vi "Target_9.vi"   [LabVIEW 2020]
uses:
  <vilib>/Platform/TimedLoop/XDataNode/timing_clust.ctl
  <vilib>/Platform/TimedLoop/XDataNode/nitl_modes.ctl
  <vilib>/Platform/TimedLoop/XDataNode/wakeup.ctl
  <vilib>/Platform/TimedLoop/XDataNode/XDataNode.xnode
  <vilib>/Platform/TimedLoop/XDataNode/XDNodeRunTimeDep.lvlib
  <vilib>/measure/NI_MABase.lvlib
types:
  T1 = typedef "XDNodeRunTimeDep.lvlib/timing_clust.ctl" = cluster{"Expected End [f-1]":u64, "Actual End [f-1]":u64, "Finished Late? [f-1]":bool, "Expected End [i-1]":u64, "Actual End [i-1]":u64, "Finished Late? [i-1]":bool, "Expected Start [i]":u64, "Actual Start [i]":u64, "Expected Start [f]":u64, "Actual Start [f]":u64, "Source Name":string, "Structure Name":string, "Period":i64, "Deadline":i64, "Offset":i64, "Start":i64, "Priority":i32, "Timeout":i32, "Mode":T2, "Wakeup Reason":T3, "Error":errorcluster, "Source Type":string, "Secondary Source Type":string, "Global End Time":u64, "Global Start Time":u64, "Frame Duration":u64, "Iteration Duration":u64, "Assigned CPU":i32, "I/O Scan Engine Mode":u32}
  T2 = typedef "XDNodeRunTimeDep.lvlib/nitl_modes.ctl" = enum32{"No Change", "Process missed periods, maintain original phase", "Discard missed periods, maintain original phase", "Process missed periods, ignore original phase", "Discard missed periods, ignore original phase"}
  T3 = typedef "XDNodeRunTimeDep.lvlib/wakeup.ctl" = enum32{"Normal", "Aborted", "Asynchronous wakeup", "Timing source error", "Timed loop error", "Timeout"}
  T4 = enum16{"Sine Wave", "Triangle Wave", "Square Wave", "Sawtooth Wave"}
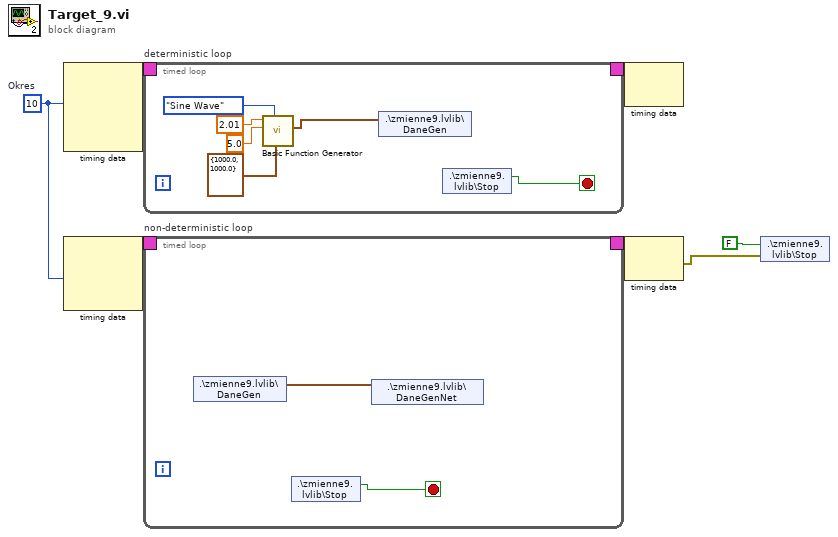
[diagram p0: block diagram]
diagram:
  w3 = i64 10  # Okres
  n1 = node-c288 ("Input Node")(w3) -> (w7:T1)  [unwired: 3 in]
  n2 = node-c288 ("Input Node")(w3) -> (w5:T1)  [unwired: 2 in]
  n3 = timed-loop "deterministic loop" {
    timing: w7 -> [_]
    timing-out: [_] -> w6
    stop <- w9 stop-if-true
    n4 = call <vilib>:"Basic Function Generator.vi"("sampling info"=cluster{"Fs":dbl, "#s":dbl} {"Fs"=1000.0, "#s"=1000.0}, "signal type"=T4."Sine Wave", "amplitude"=5.0, "frequency"=2.01) -> ("signal out"=w8:waveform(dbl))  [unwired: 5 in, 2 out]
    n5 = shared-variable ".\\zmienne9.lvlib\\DaneGen"(w8) -> ()  [unwired: 1 in, 1 out]
    n6 = shared-variable ".\\zmienne9.lvlib\\Stop"() -> (w9:bool)  [unwired: 1 in, 1 out]
  }
  n7 = timed-loop "non-deterministic loop" {
    timing: w5 -> [_]
    timing-out: [_] -> w4
    stop <- w17 stop-if-true
    n8 = shared-variable ".\\zmienne9.lvlib\\DaneGen"() -> (w16:waveform(dbl))  [unwired: 1 in, 1 out]
    n9 = shared-variable ".\\zmienne9.lvlib\\Stop"() -> (w17:bool)  [unwired: 1 in, 1 out]
    n10 = shared-variable ".\\zmienne9.lvlib\\DaneGenNet"(w16) -> ()  [unwired: 1 in, 1 out]
  }
  n11 = node-c288 ("Output Node")(w6) -> ()  [unwired: 1 out]
  n12 = node-c288 ("Output Node")(w4) -> (w1:errorcluster)
  n13 = shared-variable ".\\zmienne9.lvlib\\Stop"(FALSE ("Stop"), error in=w1) -> ()  [unwired: 1 out]
